vi "Close Account.vi"(8 "error in":errorcluster, 11 "Account info":T1) -> (0 "error out":errorcluster)   [LabVIEW 2014]
uses:
  Account Info.ctl
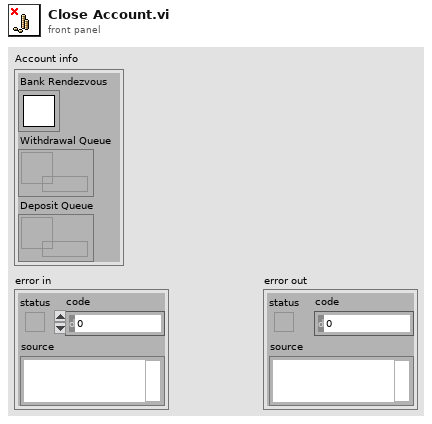
[diagram p1: front panel]
types:
  T1 = typedef "Account Info.ctl" = cluster{"Bank Rendezvous":T2, "Withdrawal Queue":refnum<queue>, "Deposit Queue":refnum<queue>}
  T2 = typedef "Rendezvous RefNum" = refnum<k1>
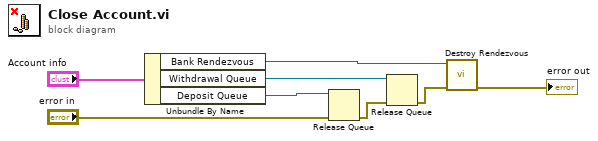
[diagram p0: block diagram]
diagram:
  n1 = Unbundle By Name("Account info") -> ("Bank Rendezvous"=w7:T2, "Withdrawal Queue"=w4:refnum<queue>, "Deposit Queue"=w6:refnum<queue>)
  n2 = Release Queue(queue=w6, error in (no error)="error in") -> (error out=w5:errorcluster)  [unwired: 1 in, 2 out]
  n3 = Release Queue(queue=w4, error in (no error)=w5) -> (error out=w3:errorcluster)  [unwired: 1 in, 2 out]
  n4 = call <vilib>:"Destroy Rendezvous.vi"("error in (no error)"=w3, "rendezvous"=w7) -> ("error out"=→"error out":errorcluster)  [unwired: 4 in, 1 out]
